vi "Calibration.vi"() -> ()   [LabVIEW 2013]
uses:
  lib/Calibration/Actuator Controls.ctl
  lib/Apps/On Off Button.ctl
  lib/Calibration/Calibration Readings.ctl
  lib/Calibration/CalibrationRampState.ctl
  lib/Calibration/SquareWaveRampState.ctl
  lib/Data Access Objects/Autobalance/Autobalance Control Parameters.ctl
  lib/Calibration/Cal Autobalance State.ctl
  lib/Apps/Yes No Button.ctl
  lib/Autobalance/Autobalance Stage.ctl
  lib/Calibration/Cal Autobalance Loop States.ctl
  lib/Autobalance/Autobalance State.ctl
  Test Utilities/DAQ Read Actions.ctl
  lib/Autobalance/Autobalance Status Data.ctl
  lib/Autobalance/Autobalance Data Point.ctl
  lib/Data Access Objects/Metadata/LBCB Number.ctl
  <vilib>/DAQmx/write.llb/DAQmx Write (Analog 1D DBL NChan 1Samp).vi
  <vilib>/DAQmx/miscellaneous.llb/DAQmx Fill In Error Info.vi
panel:
  out "Cal Sensor":dbl[](array[numeric])
  out "Cal Sensor GUI":dbl[](array[numeric]) caption="Cal Sensor"
  out "Servo Error Reading GUI":dbl[](array[numeric])=[-0.045613668785055836, 0.05618794485593462, -0.029714015687887337, -2.1182198949074764, 0.2302475954600103, 0.1361257374672665] caption="Servo Error \nReading"
  out "Load Cell \nReading  GUI":dbl[](array[numeric])=[0.004815892305044922, 0.021102771948247747, 0.11524760557242354, -0.004639114097545322, -0.030749291237820664, 0.2506269888196334] caption="Load Cell \nReading"
  out "LVDT Reading  GUI":dbl[](array[numeric])=[-0.007330159215639922, -0.035690290111210145, 0.0164473634355215, 0.754492764389709, -0.07873676501809232, -0.046523640832661604] caption="LVDT Reading"
  in  "Control Type":enum32{"Set", "Ramp", "Square", "Autobalance"}(tab)=enum."Autobalance"
  in  "Set Control":cluster{"Set":bool, "Actuator Controls":T1} {"Actuator Controls"."Actuator Z2" min=-10.0 max=10.0 step=0.1 scale=-10.0..10.0; "Actuator Controls"."Actuator Z3" min=-10.0 max=10.0 step=0.1 scale=-10.0..10.0; "Actuator Controls"."Actuator X2" min=-10.0 max=10.0 step=0.1 scale=-10.0..10.0; "Actuator Controls"."Actuator Y1" min=-10.0 max=10.0 step=0.1 scale=-10.0..10.0; "Actuator Controls"."Actuator Z1" min=-10.0 max=10.0 step=0.1 scale=-10.0..10.0; "Actuator Controls"."Actuator X1" min=-10.0 max=10.0 step=0.1 scale=-10.0..10.0}
  in  "Ramp Control":T2={"Ramp Time\n(millseconds)"=30.0, "No. of Steps"=100, "Ramp"=FALSE, "Actuator Controls"={"Actuator X1"=0.0, "Actuator X2"=0.0, "Actuator Y1"=0.0, "Actuator Z1"=0.0, "Actuator Z2"=0.0, "Actuator Z3"=0.0}} {"Actuator Controls"."Actuator Z2" min=-10.0 max=10.0 step=0.1 scale=-10.0..10.0; "Actuator Controls"."Actuator Z3" min=-10.0 max=10.0 step=0.1 scale=-10.0..10.0; "Actuator Controls"."Actuator X2" min=-10.0 max=10.0 step=0.1 scale=-10.0..10.0; "Actuator Controls"."Actuator Y1" min=-10.0 max=10.0 step=0.1 scale=-10.0..10.0; "Actuator Controls"."Actuator Z1" min=-10.0 max=10.0 step=0.1 scale=-10.0..10.0; "Actuator Controls"."Actuator X1" min=-10.0 max=10.0 step=0.1 scale=-10.0..10.0}
  in  "Ramp State":T3
  out "Number of Samples":i32=1031
  out "High Square":dbl=0.0003013857302646694
  out "Low Square":dbl=0.0003106730021702475
  in  "Square State":T4
  in  "Square Control":T5={"Hold Time\n(milliseconds)"=12000, "No. of\n Iterations"=20, "Run"=FALSE, "Actuator Controls"={"Actuator X1"=0.0, "Actuator X2"=0.0, "Actuator Y1"=0.0, "Actuator Z1"=0.2, "Actuator Z2"=0.0, "Actuator Z3"=0.0}} {"Actuator Controls"."Actuator Z2" min=-10.0 max=10.0 step=0.1 scale=-10.0..10.0; "Actuator Controls"."Actuator Z3" min=-10.0 max=10.0 step=0.1 scale=-10.0..10.0; "Actuator Controls"."Actuator X2" min=-10.0 max=10.0 step=0.1 scale=-10.0..10.0; "Actuator Controls"."Actuator Y1" min=-10.0 max=10.0 step=0.1 scale=-10.0..10.0; "Actuator Controls"."Actuator Z1" min=-10.0 max=10.0 step=0.1 scale=-10.0..10.0; "Actuator Controls"."Actuator X1" min=-10.0 max=10.0 step=0.1 scale=-10.0..10.0}
  in  "course":u32=2500
  in  "fine":i32=100
  out "Square Index":i32=3
  in  "Autobalance":bool
  in  "Error Tolerance":dbl=0.005
  out "Cal Autobalance State":T6
  in  "Autobalance \nControl Parameters":T9={"Number of Samples"=30, "Delay After Cmd"=50, "Maximum Command"=8.5, "1/4 Linear Range"=0.2}
  out "Autobalance Loop State":T10 caption="State"
  out "Autobalance State Out":T11
  in  "Zoom Type":T12(ring)=enum."Lower Edge"
  in  "Restore":bool
  in  "Zoom In":bool
  in  "Readings":T13
  in  "Actuator":i32(listbox)=3
  out "Readings":T14(graph)={"Average[0]"=-0.007330159215639922, "Average[1]"=-0.035690290111210145, "Average[2]"=0.0164473634355215, "Average[3]"=0.754492764389709, "Average[4]"=-0.07873676501809232, "Average[5]"=-0.046523640832661604, "Average[6]"=0.0, "Average[7]"=0.0, "Average[8]"=0.0}
  in  "Logging":T15
  out "Command \nVoltage":dbl[](array[numeric])
  in  "Log File Path":path=path "C:/Documents and Settings/mbletzin/Desktop/CalVolts.txt"
  out "Control Voltage":dbl[](array[numeric])
  in  "rate":dbl=100.0
  in  "samples per \nchannel":i32=30 caption="samples per channel"
  out "Servo Error Reading":dbl[](array[numeric])=[-0.045067125531769704, 0.05668122915132235, -0.02948210200083762, -2.1175081409061565, 0.230346235434936, 0.13661629420139546]
  in  "Command Voltage Task":refnum<k21>="Command Voltage"
  in  "Readings Task":refnum<k21>="All Readings"
  out "Read error out":errorcluster
  out "Write error out":errorcluster
  in  "Read error in (no error)":errorcluster
  out "Load Cell \nReading":dbl[](array[numeric])=[0.004986511517158722, 0.021102771948253347, 0.11523427762419364, -0.004596456436788376, -0.03101586222110612, 0.24965138792681876]
  out "LVDT Reading":dbl[](array[numeric])=[-0.007431458122470593, -0.03581289816268755, 0.016426039174719534, 0.7542049018799244, -0.07857947210067343, -0.04675023078564846]
  in  "Quit":bool
  # "LBCB CALIBRATION PROGRAM"
  # "Sample Window Size"
  # "msec"
  # "deleted\nsamples"
  # "Is Balanced"
  # "State"
  # "(Volts)"
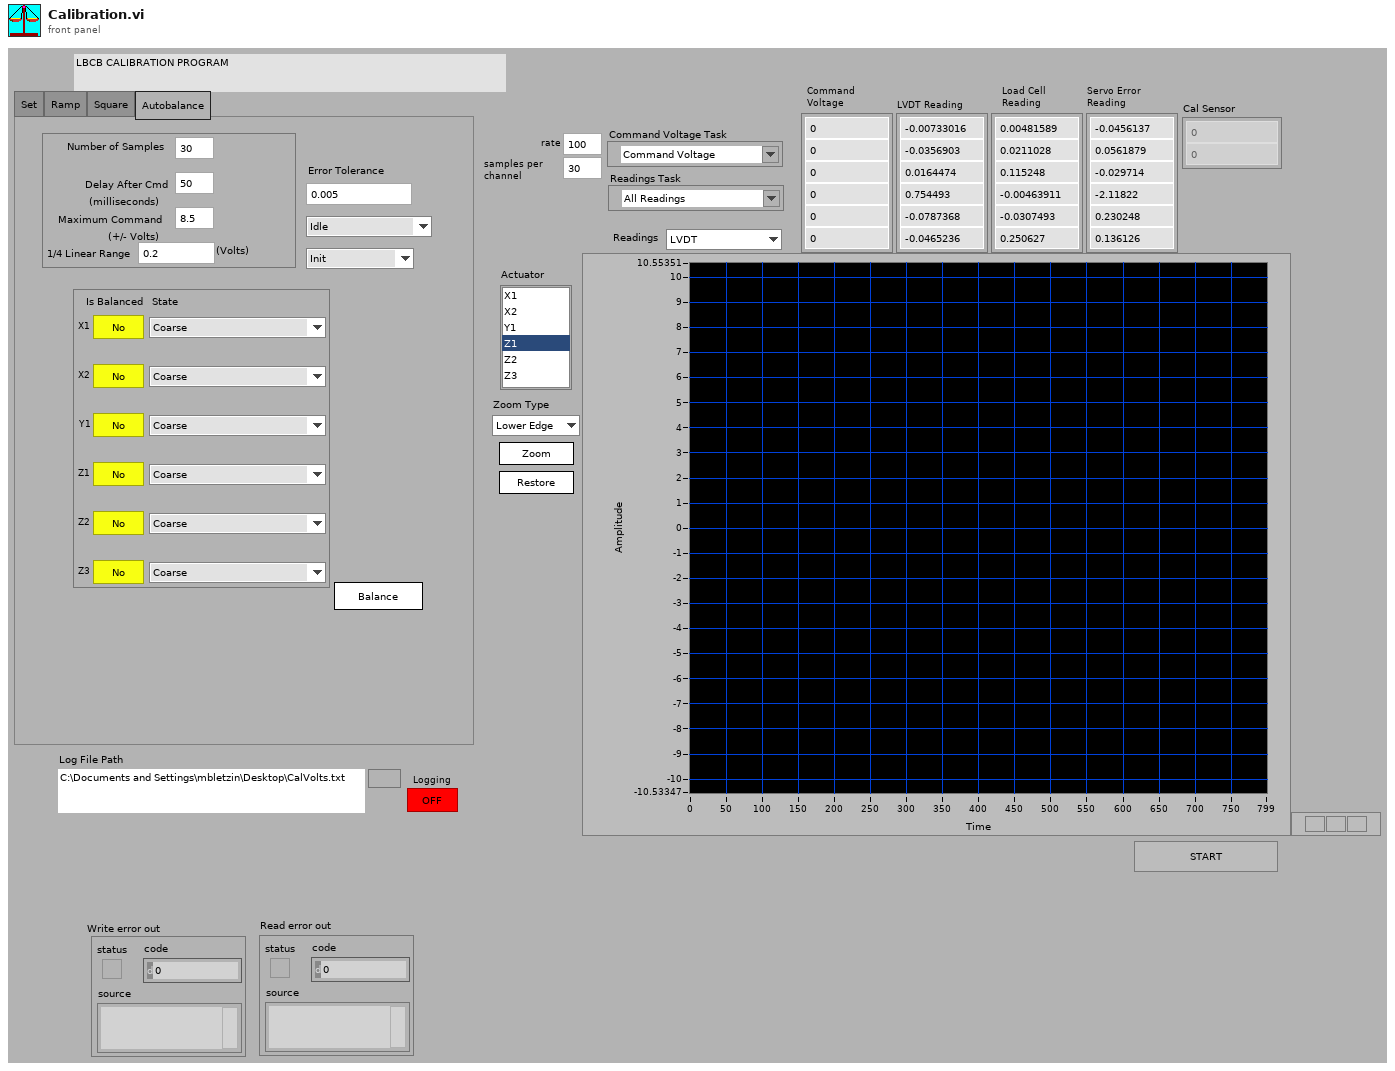
[diagram p1: front panel]
types:
  T1 = typedef "Actuator Controls.ctl" = cluster{"Actuator X1":dbl, "Actuator X2":dbl, "Actuator Y1":dbl, "Actuator Z1":dbl, "Actuator Z2":dbl, "Actuator Z3":dbl}
  T2 = cluster{"Ramp Time\n(millseconds)":dbl, "No. of Steps":i32, "Ramp":bool, "Actuator Controls":T1}
  T3 = typedef "CalibrationRampState.ctl" = enum16{"Idle", "Start Ramp", "Ramping", "Stopping"}
  T4 = typedef "SquareWaveRampState.ctl" = enum16{"Idle", "Start Wave", "High", "Low", "Stop"}
  T5 = cluster{"Hold Time\n(milliseconds)":i32, "No. of\n Iterations":i32, "Run":bool, "Actuator Controls":T1}
  T6 = typedef "Cal Autobalance State.ctl" = cluster{"X1 IsBalanced":T7, "X1 State":T8, "X2 IsBalanced":T7, "X2 State":T8, "Y1 IsBalanced":T7, "Y1 State":T8, "Z1 IsBalanced":T7, "Z1 State":T8, "Z2 IsBalanced":T7, "Z2 State":T8, "Z3 IsBalanced":T7, "Z3 State":T8}
  T7 = typedef "Yes No Button.ctl" = bool
  T8 = typedef "Autobalance Stage.ctl" = enum16{"Coarse", "Fine", "Backing Up", "Done"}
  T9 = typedef "Autobalance Control Parameters.ctl" = cluster{"Number of Samples":i32, "Delay After Cmd":i32, "Maximum Command":dbl, "1/4 Linear Range":dbl}
  T10 = typedef "Cal Autobalance Loop States.ctl" = enum16{"Idle", "Start Balancing", "Balancing", "Stop"}
  T11 = typedef "Autobalance State.ctl" = enum16{"Init", "Send High ", "Wait High", "Read High Start", "Read High", "Send Low", "Wait Low", "Read Low Start", "Read Low", "Publish", "Calculate", "Done"}
  T12 = enum16{"Full", "Upper Half", "Upper Edge", "Lower Half", "Lower Edge"}
  T13 = typedef "Calibration Readings.ctl" = enum16{"LVDT", "Load Cell", "Servo Errors"}
  T14 = cluster{"Average[0]":dbl, "Average[1]":dbl, "Average[2]":dbl, "Average[3]":dbl, "Average[4]":dbl, "Average[5]":dbl, "Average[6]":dbl, "Average[7]":dbl, "Average[8]":dbl}
  T15 = typedef "On Off Button.ctl" = bool
  T16 = enum8{"Enabled", "Disabled", "Disabled and Grayed Out"}
  T17 = typedef "DAQ Read Actions.ctl" = enum16{"Start", "Read", "Stop"}
  T18 = typedef "Autobalance Status Data.ctl" = cluster{"IsBalanced":T7, "Autobalance Stage":T8, "High":T19, "Low":T19, "Balanced \nCmd":dbl}
  T19 = typedef "Autobalance Data Point.ctl" = cluster{"cCmd":dbl, "cServo":dbl, "pCmd":dbl, "pServo":dbl}
  T20 = typedef "LBCB Number.ctl" = enum16{"LBCB1", "LBCB2"}
  T21 = cluster{"Average[0]":dbl, "Average[1]":dbl, "Average[2]":dbl, "Average[3]":dbl, "Average[4]":dbl, "Average[5]":dbl, "Average[6]":dbl, "Average[7]":dbl, "Average[8]":dbl}[]
  T22 = enum16{"open", "replace", "create", "open or create", "replace or create", "replace or create with confirmation"}
  T23 = cluster{"Servo Error Reading[0]":dbl, "Servo Error Reading[1]":dbl, "Servo Error Reading[2]":dbl, "Servo Error Reading[3]":dbl, "Servo Error Reading[4]":dbl, "Servo Error Reading[5]":dbl, "Servo Error Reading[6]":dbl, "Servo Error Reading[7]":dbl, "Servo Error Reading[8]":dbl}
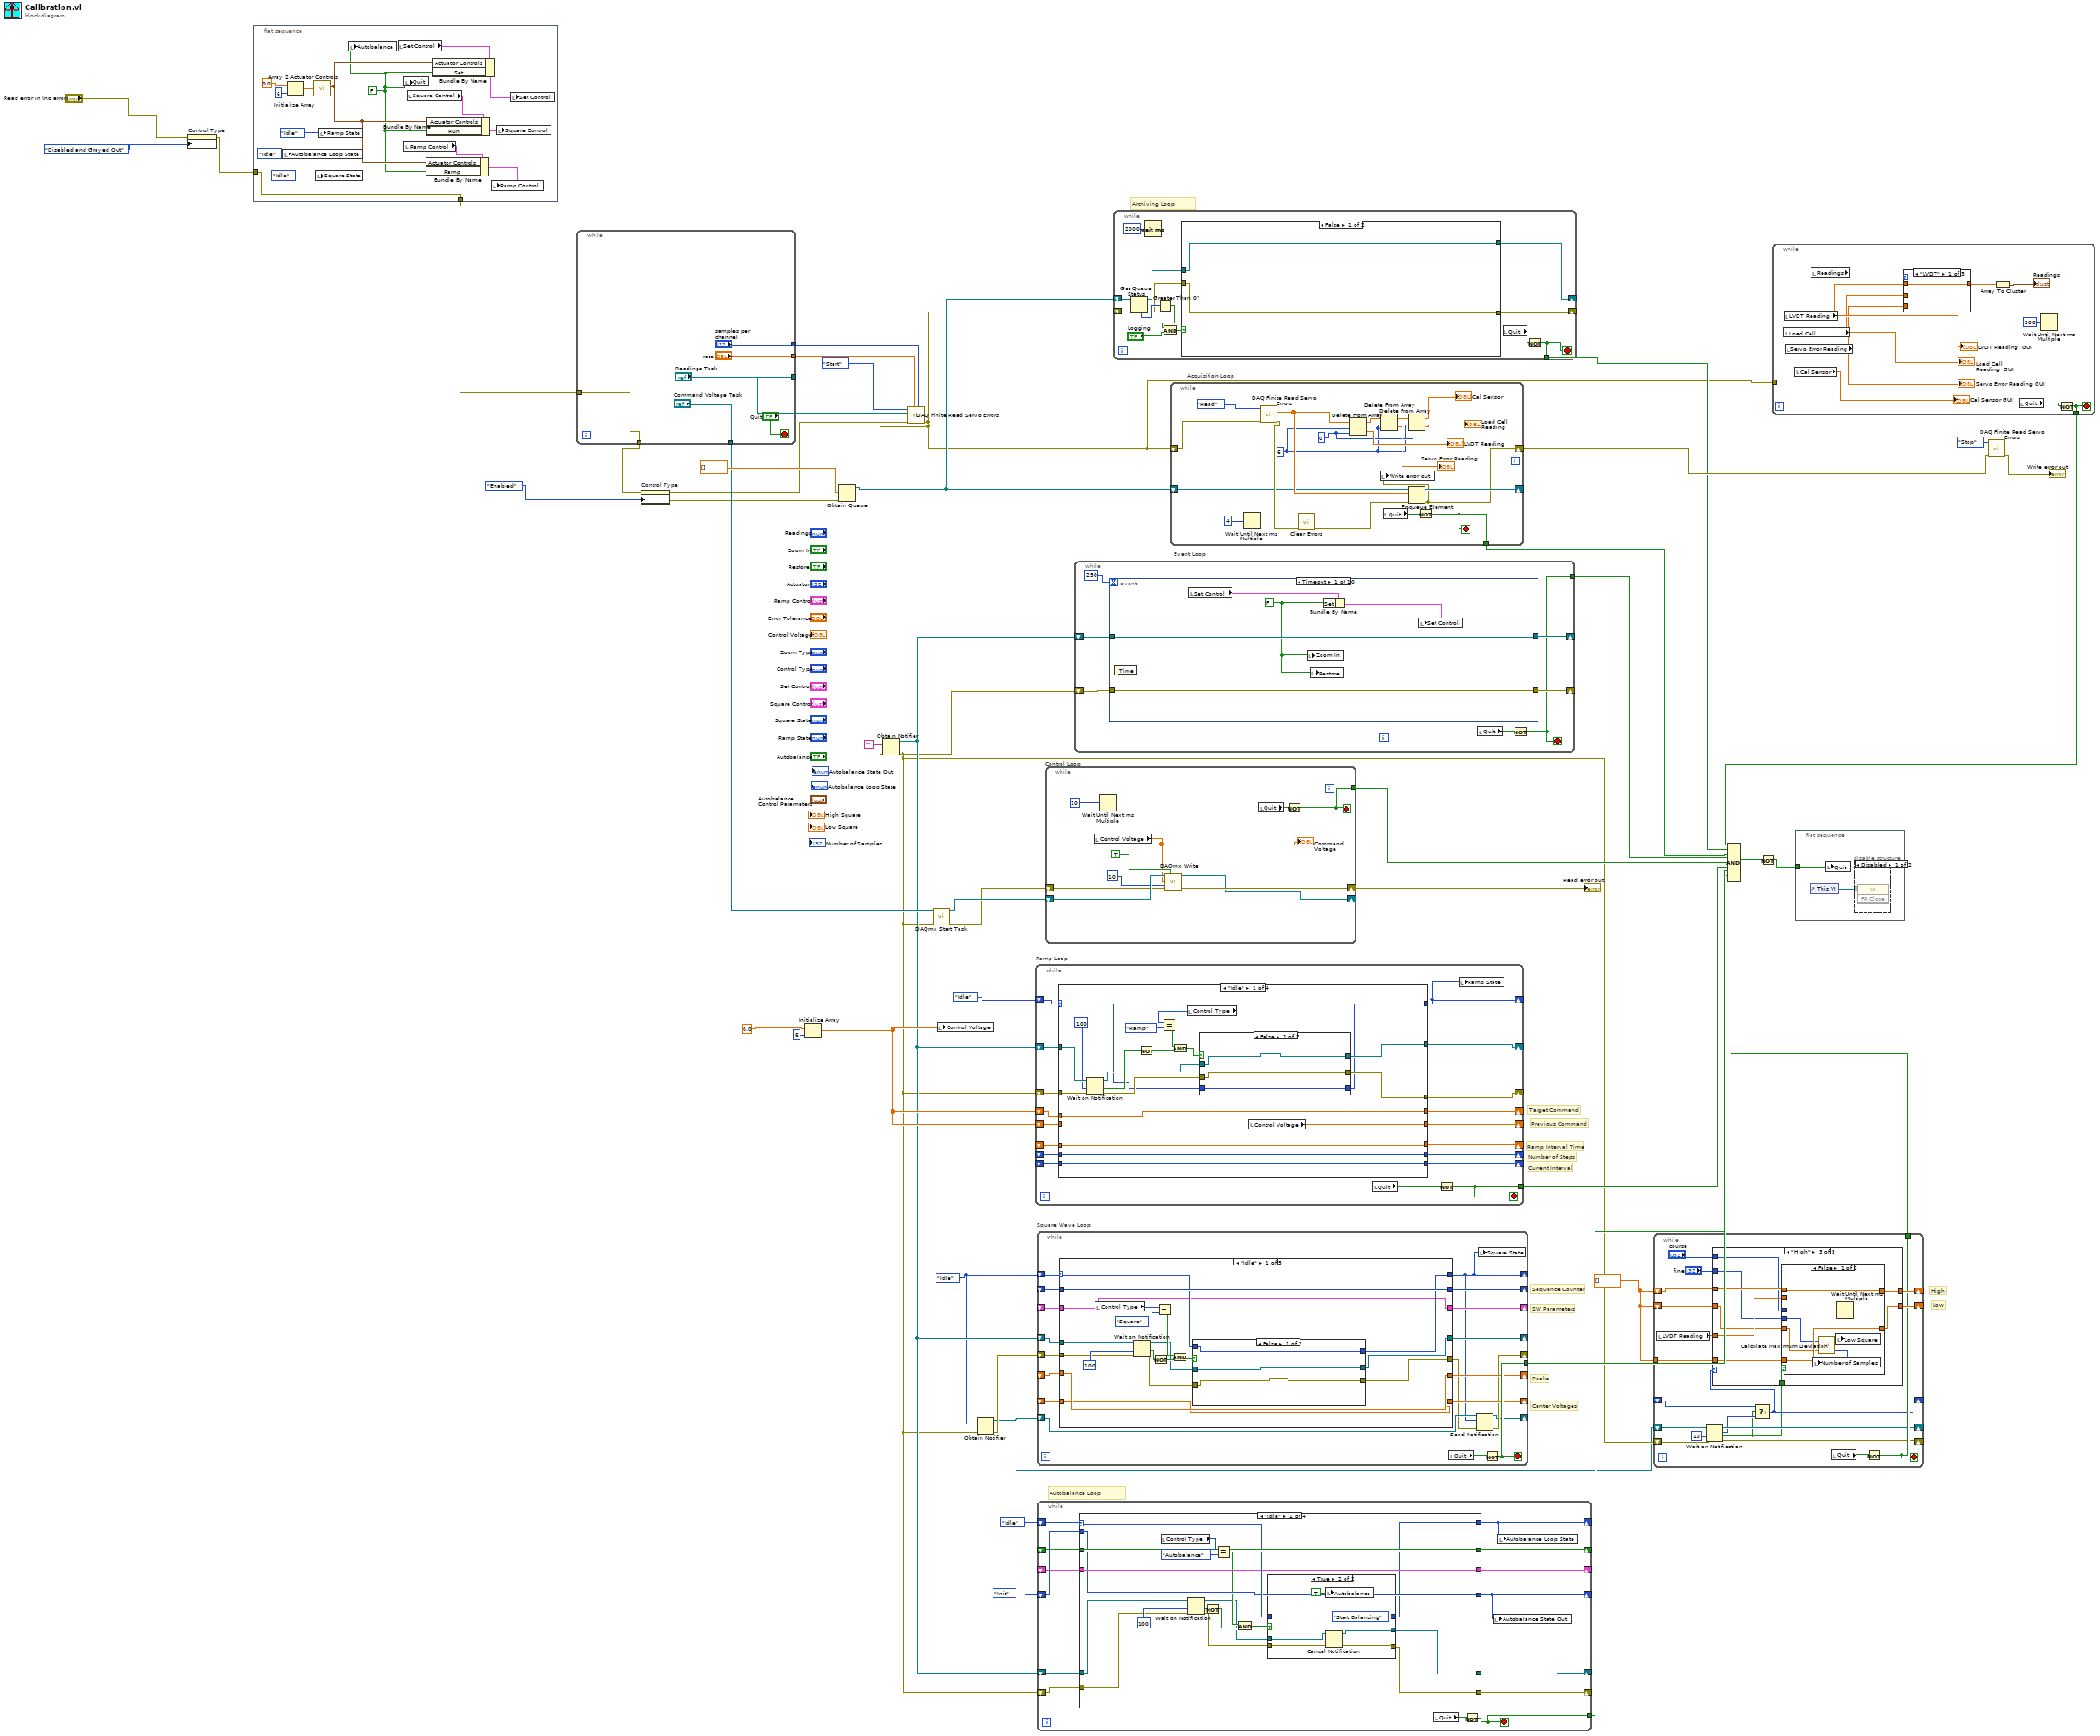
[diagram p0: block diagram]
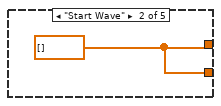
[diagram p5: hidden frame]
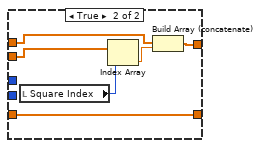
[diagram p6: hidden frame]
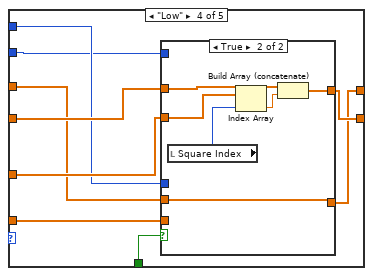
[diagram p7: hidden frame]
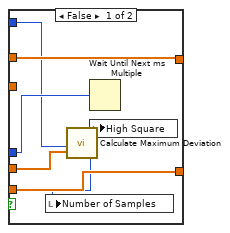
[diagram p8: hidden frame]
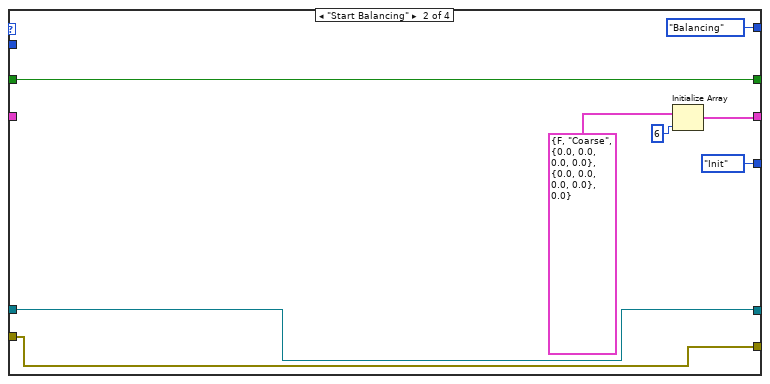
[diagram p11: hidden frame]
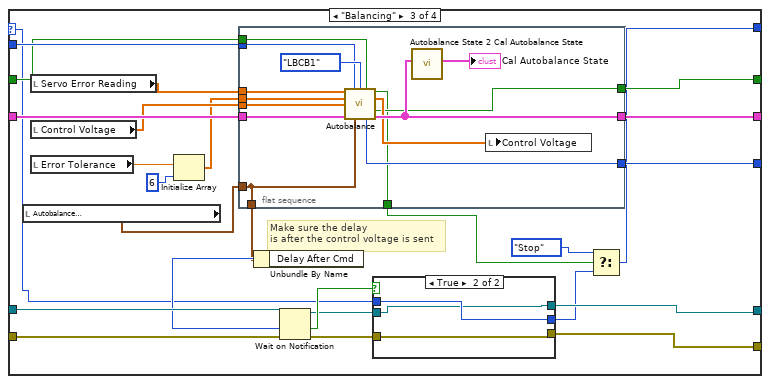
[diagram p12: hidden frame]
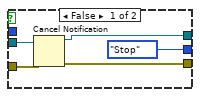
[diagram p13: hidden frame]
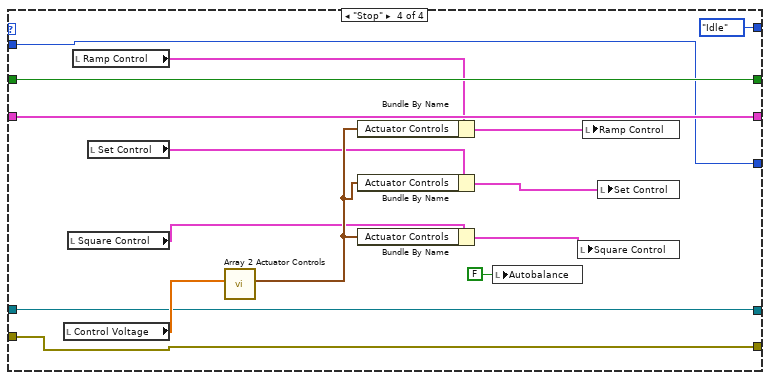
[diagram p14: hidden frame]
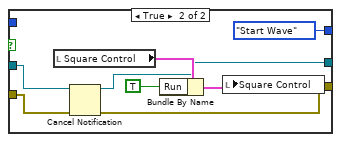
[diagram p15: hidden frame]
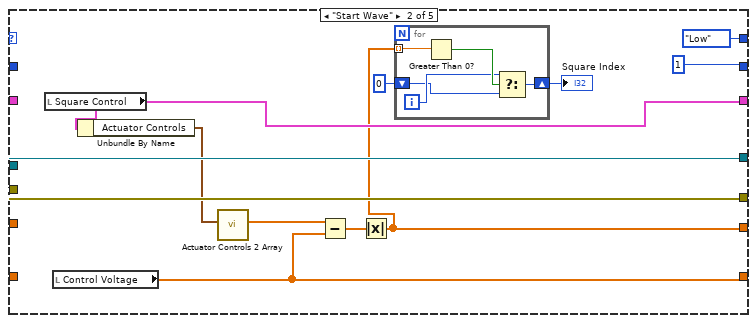
[diagram p16: hidden frame]
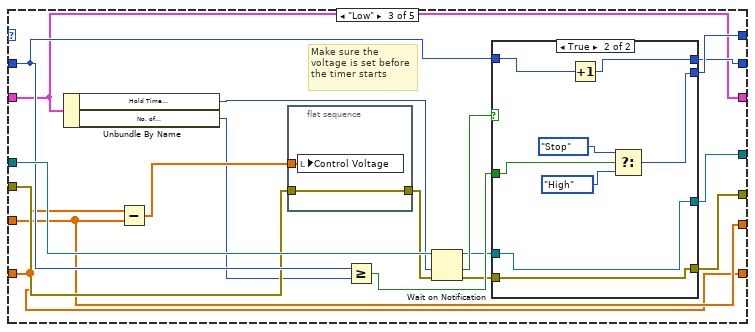
[diagram p17: hidden frame]
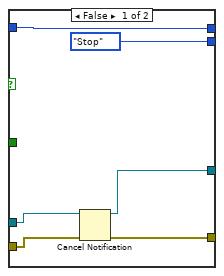
[diagram p18: hidden frame]
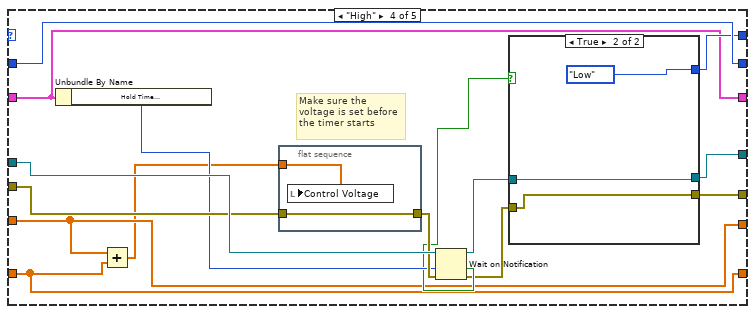
[diagram p19: hidden frame]
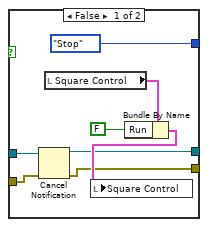
[diagram p20: hidden frame]
diagram:
  w5 = dbl[] []
  w4 = SquareWaveRampState."Idle" ("Square State")
  # "Low"
  # "High"
  # "Autobalance Loop"
  # "Peaks"
  # "Center Voltages"
  # "Archiving Loop"
  # "SW Parameters"
  # "Sequence Counter"
  # "Previous Command"
  # "Target Command"
  # "Ramp Interval Time"
  # "Number of Steps"
  # "Current Interval"
  n1 = property on="Control Type" class="TabCtl (strict)"(error in="Read error in (no error)", "DisabledEnum"=T16."Disabled and Grayed Out" ("Disabled")) -> (error out=w12:errorcluster)  [unwired: 1 in, 1 out]
  n2 = flat-sequence {
    tunnel: w12 -> [w50]
    tunnel: [w50] -> w15
    frame #0 {
      w46 = FALSE
      n3 = local write "Autobalance Loop State"(Cal_Autobalance_Loop_States."Idle" ("Autobalance Loop State")) -> ()
      n4 = Initialize Array(0.0 ("element"), 6 ("dimension size")) -> (w58:dbl[])
      n5 = call "Array 2 Actuator Controls.vi"("Array"=w58) -> ("Actuator Controls"=w51:T1)  [unwired: 10 in]
      n6 = local write "Square State"(SquareWaveRampState."Idle" ("Square State")) -> ()
      n7 = local write "Ramp State"(CalibrationRampState."Idle" ("Ramp State")) -> ()
      n8 = local write "Autobalance"(w46) -> ()
      n9 = local read "Set Control"() -> (w54:cluster{"Set":bool, "Actuator Controls":T1})
      n10 = local write "Quit"(w46) -> ()
      n11 = local read "Ramp Control"() -> (w52:T2)
      n12 = local read "Square Control"() -> (w56:T5)
      n13 = Bundle By Name(cluster=w52, "Actuator Controls"=w51, "Ramp"=w46) -> (w53:T2)
      n14 = Bundle By Name(cluster=w56, "Actuator Controls"=w51, "Run"=w46) -> (w57:T5)
      n15 = Bundle By Name(cluster=w54, "Actuator Controls"=w51, "Set"=w46) -> (w55:cluster{"Set":bool, "Actuator Controls":T1})
      n16 = local write "Ramp Control"(w53) -> ()
      n17 = local write "Square Control"(w57) -> ()
      n18 = local write "Set Control"(w55) -> ()
    }
  }
  n19 = while {
    tunnel: [w61] -> w11
    tunnel: ["samples per \nchannel"] -> w26
    tunnel: ["rate"] -> w25
    tunnel: ["Readings Task"] -> w24
    tunnel: ["Command Voltage Task"] -> w23
    tunnel: w15 -> [w61]
    stop <- "Quit" stop-if-true
  }
  n20 = property on="Control Type" class="TabCtl (strict)"(error in=w11, "DisabledEnum"=T16."Enabled" ("Disabled")) -> (error out=w10:errorcluster)  [unwired: 1 in, 1 out]
  n21 = Initialize Array(0.0 ("element"), 6 ("dimension size")) -> (w22:dbl[])
  n22 = Obtain Queue(element data type=dbl[] [], error in (no error)=w10) -> (queue out=w30:refnum<queue>)  [unwired: 3 in, 2 out]
  n23 = call "DAQ Finite Read Servo Errors.vi"("samples per channel"=w26, "rate"=w25, "error in"=w10, "task/channels in"=w24, "Action"=DAQ_Read_Actions."Start") -> ("error out"=w8:errorcluster)  [unwired: 6 out]
  n24 = Obtain Notifier(notification data type="", error in (no error)=w8) -> (notifier out=w16:refnum<notifier>, error out=w3:errorcluster)  [unwired: 2 in, 1 out]
  n25 = call <vilib>:"DAQmx Start Task.vi"("task/channels in"=w23, "error in"=w3) -> ("task out"=w45:refnum<k21>, "error out"=w20:errorcluster)  [unwired: 12 out]
  n26 = local write "Control Voltage"(w22) -> ()
  n27 = Obtain Notifier(notification data type=w4, error in (no error)=w3) -> (notifier out=w1:refnum<notifier>, error out=w2:errorcluster)  [unwired: 2 in, 1 out]
  n28 = while "Ramp Loop" {
    shift-right: [w67] -> _
    shift-left: CalibrationRampState."Idle" ("Ramp State") -> [w84]
    shift-right: [w81] -> _
    shift-left: w16 -> [w83]
    shift-right: [w80] -> _
    shift-left: w3 -> [w82]
    shift-right: [w79] -> _
    shift-left: _ -> [w71]
    shift-right: [w77] -> _
    shift-left: _ -> [w72]
    shift-right: [w78] -> _
    shift-left: _ -> [w73]
    shift-right: [w76] -> _
    shift-left: w22 -> [w74]
    shift-right: [w75] -> _
    shift-left: w22 -> [w70]
    tunnel: [w68] -> w32
    stop <- w68 stop-if-true
    n29 = case shown="\"Idle\"" w84 {
      selector: w84 -> [w85 _ w139 _]
      tunnel: w83 -> [w104 w125 w138 w173]
      tunnel: w82 -> [w103 w126 w134 w168]
      tunnel: [w87 w125 w132 w173] -> w81
      tunnel: [w88 w126 w128 w168] -> w80
      tunnel: [w86 CalibrationRampState."Ramping" ("f") w129 CalibrationRampState."Idle" ("f")] -> w67
      tunnel: [w99 w122 w147 w171] -> w79
      tunnel: [w97 0 w146 w169] -> w78
      tunnel: [w98 w120 w140 w170] -> w77
      tunnel: [w101 w119 w136 w174] -> w76
      tunnel: [w100 w116 w137 w175] -> w75
      tunnel: w74 -> [_ w119 w136 _]
      tunnel: w73 -> [w97 _ w141 w169]
      tunnel: w72 -> [w98 _ w140 w170]
      tunnel: w71 -> [w99 _ w147 w171]
      tunnel: w70 -> [w100 _ w137 w175]
      frame "Idle" {
        n30 = Wait on Notification(notifier=w104, timeout in ms (-1)=100, error in (no error)=w103) -> (notifier out=w90:refnum<notifier>, timed out?=w96:bool, error out=w89:errorcluster)  [unwired: 1 in, 1 out]
        n31 = Not(x=w96) -> (.not. x?=w91:bool)
        n32 = local read "Control Type"() -> (w95:enum32{"Set", "Ramp", "Square", "Autobalance"})
        n33 = Equal?(x=w95, y=enum32{"Set", "Ramp", "Square", "Autobalance"}."Ramp") -> (x = y?=w93:bool)
        n34 = And(x=w93, y=w91) -> (x .and. y?=w94:bool)
        n35 = case shown="False" w94 {
          tunnel: w90 -> [w107 w112]
          tunnel: w89 -> [w106 w111]
          tunnel: [w106 w109] -> w88
          tunnel: [w107 w110] -> w87
          tunnel: [w105 CalibrationRampState."Start Ramp" ("f")] -> w86
          tunnel: w85 -> [w105 _]
          frame False {
          }
          frame True {
            n36 = local read "Ramp Control"() -> (w115:T2)
            n37 = Bundle By Name(cluster=w115, "Ramp"=TRUE) -> (w114:T2)
            n38 = local write "Ramp Control"(w114) -> ()
            n39 = Cancel Notification(0:w112, 3:w111) -> (8:w110:refnum<notifier>, 11:w109:errorcluster)  [unwired: 1 out]
          }
        }
        n40 = local read "Control Voltage"() -> (w101:dbl[])
      }
      frame "Start Ramp" {
        n41 = local read "Ramp Control"() -> (w118:T2)
        n42 = Unbundle By Name(w118) -> ("Ramp Time\n(millseconds)"=w123:dbl, "No. of Steps"=w120:i32, "Actuator Controls"=w117:T1)
        n43 = call "Actuator Controls 2 Array.vi"("Actuator Controls"=w117) -> ("Array"=w116:dbl[])  [unwired: 10 in]
        n44 = Divide(x=w123, y=w120) -> (x/y=w122:dbl)
      }
      frame "Ramping" {
        n45 = Increment(x=w141) -> (x+1=w146:i32)
        n46 = Subtract(x=w137, y=w136) -> (x-y=w145:dbl[])
        n47 = Less?(x=w140, y=w141) -> (x < y?=w142:bool)
        n48 = Divide(x=w146, y=w140) -> (x/y=w144:dbl)
        n49 = case shown="True" w142 {
          tunnel: w145 -> [w162 _]
          tunnel: w144 -> [w161 _]
          tunnel: [w158 w163] -> w143
          tunnel: w139 -> [w159 _]
          tunnel: [w159 CalibrationRampState."Stopping" ("Ramp State")] -> w127
          tunnel: w137 -> [_ w163]
          tunnel: w136 -> [w157 _]
          frame False {
            n50 = Multiply(x=w162, y=w161) -> (x*y=w160:dbl[])
            n51 = Add(x=w160, y=w157) -> (x+y=w158:dbl[])
          }
          frame True {
          }
        }
        n52 = Multiply(x=w147, y=1000.0) -> (x*y=w135:dbl)
        n53 = local write "Control Voltage"(w143) -> ()
        n54 = Wait on Notification(notifier=w138, timeout in ms (-1)=w135, error in (no error)=w134) -> (notifier out=w133:refnum<notifier>, timed out?=w130:bool, error out=w131:errorcluster)  [unwired: 1 in, 1 out]
        n55 = case shown="True" w130 {
          tunnel: w133 -> [w153 w156]
          tunnel: [w152 w156] -> w132
          tunnel: w131 -> [w150 w154]
          tunnel: [CalibrationRampState."Stopping" ("f") w155] -> w129
          tunnel: [w149 w154] -> w128
          tunnel: w127 -> [_ w155]
          frame False {
            n56 = Cancel Notification(0:w153, 3:w150) -> (8:w152:refnum<notifier>, 11:w149:errorcluster)  [unwired: 1 out]
          }
          frame True {
          }
        }
      }
      frame "Stopping" {
        n57 = local read "Set Control"() -> (w182:cluster{"Set":bool, "Actuator Controls":T1})
        n58 = local read "Ramp Control"() -> (w181:T2)
        n59 = local read "Square Control"() -> (w180:T5)
        n60 = local read "Control Voltage"() -> (w174:dbl[])
        n61 = local read "Ramp Control"() -> (w167:T2)
        n62 = call "Array 2 Actuator Controls.vi"("Array"=w174) -> ("Actuator Controls"=w179:T1)  [unwired: 10 in]
        n63 = Bundle By Name(cluster=w182, "Actuator Controls"=w179) -> (w178:cluster{"Set":bool, "Actuator Controls":T1})
        n64 = Bundle By Name(cluster=w181, "Actuator Controls"=w179) -> (w177:T2)
        n65 = Bundle By Name(cluster=w180, "Actuator Controls"=w179) -> (w176:T5)
        n66 = Bundle By Name(cluster=w167, "Ramp"=FALSE) -> (w166:T2)
        n67 = local write "Square Control"(w176) -> ()
        n68 = local write "Ramp Control"(w177) -> ()
        n69 = local write "Set Control"(w178) -> ()
        n70 = local write "Ramp Control"(w166) -> ()
      }
    }
    n71 = local read "Quit"() -> (w69:bool)
    n72 = Not(x=w69) -> (.not. x?=w68:bool)
    n73 = local write "Ramp State"(w67) -> ()
  }
  n74 = while "Square Wave Loop" {
    tunnel: [w199] -> w21
    shift-right: [w184] -> _
    shift-left: w2 -> [w198]
    shift-right: [w196] -> _
    shift-left: w16 -> [w197]
    shift-right: [w186] -> _
    shift-left: w4 -> [w201]
    shift-right: [w195] -> _
    shift-left: _ -> [w194]
    shift-right: [w193] -> _
    shift-left: _ -> [w191]
    shift-right: [w192] -> _
    shift-left: _ -> [w190]
    shift-right: [w189] -> _
    shift-left: _ -> [w188]
    shift-right: [w183] -> _
    shift-left: w1 -> [w187]
    stop <- w199 stop-if-true
    n75 = case shown="\"Idle\"" w201 {
      selector: w201 -> [w216 _ _ _ _]
      tunnel: w198 -> [w219 w243 w260 w296 w316]
      tunnel: [w202 w243 w249 w283 w316] -> w185
      tunnel: w197 -> [w218 w242 w263 w297 w317]
      tunnel: [w203 w242 w250 w284 w317] -> w196
      tunnel: [w215 SquareWaveRampState."Low" ("Square State") w266 w291 SquareWaveRampState."Idle" ("t")] -> w186
      tunnel: [w217 1 w264 w293 w319] -> w195
      tunnel: w194 -> [w217 _ w262 w293 w319]
      tunnel: [w213 w237 w253 w290 w314] -> w193
      tunnel: [w214 w234 w254 w289 w315] -> w192
      tunnel: w191 -> [w213 _ w253 w290 w314]
      tunnel: w190 -> [w214 _ w254 w289 w315]
      tunnel: [w212 w235 w255 w287 w318] -> w189
      tunnel: w188 -> [w212 _ w255 w287 w325]
      frame "Idle" {
        n76 = local read "Control Type"() -> (w207:enum32{"Set", "Ramp", "Square", "Autobalance"})
        n77 = Wait on Notification(notifier=w218, timeout in ms (-1)=100, error in (no error)=w219) -> (notifier out=w205:refnum<notifier>, timed out?=w210:bool, error out=w204:errorcluster)  [unwired: 1 in, 1 out]
        n78 = Not(x=w210) -> (.not. x?=w206:bool)
        n79 = Equal?(x=w207, y=enum32{"Set", "Ramp", "Square", "Autobalance"}."Square") -> (x = y?=w211:bool)
        n80 = And(x=w211, y=w206) -> (x .and. y?=w209:bool)
        n81 = case shown="False" w209 {
          tunnel: w216 -> [w223 _]
          tunnel: [w223 SquareWaveRampState."Start Wave" ("Square State")] -> w215
          tunnel: w205 -> [w222 w227]
          tunnel: w204 -> [w221 w226]
          tunnel: [w222 w225] -> w203
          tunnel: [w221 w224] -> w202
          frame False {
          }
          frame True {
            n82 = local read "Square Control"() -> (w231:T5)
            n83 = Cancel Notification(0:w227, 3:w226) -> (8:w225:refnum<notifier>, 11:w224:errorcluster)  [unwired: 1 out]
            n84 = Bundle By Name(cluster=w231, "Run"=TRUE) -> (w230:T5)
            n85 = local write "Square Control"(w230) -> ()
          }
        }
      }
      frame "Start Wave" {
        n86 = local read "Square Control"() -> (w235:T5)
        n87 = local read "Control Voltage"() -> (w237:dbl[])
        n88 = Unbundle By Name(w235) -> ("Actuator Controls"=w239:T1)
        n89 = call "Actuator Controls 2 Array.vi"("Actuator Controls"=w239) -> ("Array"=w238:dbl[])  [unwired: 10 in]
        n90 = Subtract(x=w238, y=w237) -> (x-y=w236:dbl[])
        n91 = Absolute Value(x=w236) -> (abs(x)=w234:dbl[])
        n92 = for {
          tunnel: w234 -> [w248] mode=indexing
          shift-right: [w247] -> w232
          shift-left: 0 -> [w244]
          i -> [w245]
          n93 = Greater Than 0?(x=w248) -> (x > 0?=w246:bool)
          n94 = Select(t=w245, s=w246, f=w244) -> (s? t:f=w247:i32)
        }
        "Square Index" <- w232
      }
      frame "Low" {
        # "Make sure the \nvoltage is set before\nthe timer starts"
        n95 = Unbundle By Name(w255) -> ("Hold Time\n(milliseconds)"=w256:i32, "No. of\n Iterations"=w257:i32)
        n96 = Subtract(x=w253, y=w254) -> (x-y=w258:dbl[])
        n97 = flat-sequence {
          tunnel: w260 -> [w268]
          tunnel: [w268] -> w259
          tunnel: w258 -> [w267]
          frame #0 {
            n98 = local write "Control Voltage"(w267) -> ()
          }
        }
        n99 = Greater Or Equal?(x=w262, y=w257) -> (x >= y?=w265:bool)
        n100 = Wait on Notification(notifier=w263, timeout in ms (-1)=w256, error in (no error)=w259) -> (notifier out=w252:refnum<notifier>, timed out?=w261:bool, error out=w251:errorcluster)  [unwired: 1 in, 1 out]
        n101 = case shown="True" w261 {
          tunnel: [SquareWaveRampState."Stop" ("t") w275] -> w266
          tunnel: w265 -> [_ w276]
          tunnel: w262 -> [w274 w282]
          tunnel: [w274 w281] -> w264
          tunnel: w252 -> [w272 w280]
          tunnel: w251 -> [w271 w279]
          tunnel: [w270 w280] -> w250
          tunnel: [w269 w279] -> w249
          frame False {
            n102 = Cancel Notification(0:w272, 3:w271) -> (8:w270:refnum<notifier>, 11:w269:errorcluster)  [unwired: 1 out]
          }
          frame True {
            n103 = Increment(x=w282) -> (x+1=w281:i32)
            n104 = Select(t=SquareWaveRampState."Stop", s=w276, f=SquareWaveRampState."High" ("t")) -> (s? t:f=w275:T4)
          }
        }
      }
      frame "High" {
        # "Make sure the \nvoltage is set before\nthe timer starts"
        n105 = Unbundle By Name(w287) -> ("Hold Time\n(milliseconds)"=w294:i32)
        n106 = Add(x=w289, y=w290) -> (x+y=w288:dbl[])
        n107 = flat-sequence {
          tunnel: w296 -> [w310]
          tunnel: [w310] -> w295
          tunnel: w288 -> [w309]
          frame #0 {
            n108 = local write "Control Voltage"(w309) -> ()
          }
        }
        n109 = Wait on Notification(notifier=w297, timeout in ms (-1)=w294, error in (no error)=w295) -> (notifier out=w286:refnum<notifier>, timed out?=w292:bool, error out=w285:errorcluster)  [unwired: 1 in, 1 out]
        n110 = case shown="True" w292 {
          tunnel: [SquareWaveRampState."Stop" ("t") SquareWaveRampState."Low" ("t")] -> w291
          tunnel: w286 -> [w301 w307]
          tunnel: w285 -> [w300 w306]
          tunnel: [w299 w307] -> w284
          tunnel: [w298 w306] -> w283
          frame False {
            n111 = Cancel Notification(0:w301, 3:w300) -> (8:w299:refnum<notifier>, 11:w298:errorcluster)  [unwired: 1 out]
            n112 = local read "Square Control"() -> (w304:T5)
            n113 = Bundle By Name(cluster=w304, "Run"=FALSE) -> (w302:T5)
            n114 = local write "Square Control"(w302) -> ()
          }
          frame True {
          }
        }
      }
      frame "Stop" {
        n115 = local read "Ramp Control"() -> (w324:T2)
        n116 = local read "Set Control"() -> (w322:cluster{"Set":bool, "Actuator Controls":T1})
        n117 = local read "Square Control"() -> (w313:T5)
        n118 = call "Array 2 Actuator Controls.vi"("Array"=w314) -> ("Actuator Controls"=w326:T1)  [unwired: 10 in]
        n119 = Bundle By Name(cluster=w325, "Actuator Controls"=w326) -> (w318:T5)
        n120 = Bundle By Name(cluster=w324, "Actuator Controls"=w326) -> (w323:T2)
        n121 = Bundle By Name(cluster=w322, "Actuator Controls"=w326) -> (w321:cluster{"Set":bool, "Actuator Controls":T1})
        n122 = Bundle By Name(cluster=w313, "Run"=FALSE) -> (w311:T5)
        n123 = local write "Control Voltage"(w314) -> ()
        n124 = local write "Square Control"(w311) -> ()
        n125 = local write "Square Control"(w318) -> ()
        n126 = local write "Ramp Control"(w323) -> ()
        n127 = local write "Set Control"(w321) -> ()
      }
    }
    n128 = local read "Quit"() -> (w200:bool)
    n129 = Send Notification(notification=w186, notifier=w187, error in (no error)=w185) -> (notifier out=w183:refnum<notifier>, error out=w184:errorcluster)
    n130 = local write "Square State"(w186) -> ()
    n131 = Not(x=w200) -> (.not. x?=w199:bool)
  }
  n132 = while {
    shift-right: [w327] -> _
    shift-left: Cal_Autobalance_Loop_States."Idle" ("Square State") -> [w340]
    shift-right: [w338] -> _
    shift-left: _ -> [w339]
    shift-right: [w328] -> _
    shift-left: Autobalance_State."Init" ("Autobalance State Out") -> [w337]
    shift-right: [w336] -> _
    shift-left: _ -> [w335]
    shift-right: [w330] -> _
    shift-left: w3 -> [w332]
    shift-right: [w331] -> _
    shift-left: w16 -> [w333]
    tunnel: [w329] -> w17
    stop <- w329 stop-if-true
    n133 = case shown="\"Idle\"" w340 {
      selector: w340 -> [w352 _ w378 _]
      tunnel: w339 -> [w357 _ w400 w436]
      tunnel: [w357 w373 w399 w436] -> w338
      tunnel: [w351 Autobalance_State."Init" ("Autobalance State Out") w398 w435] -> w328
      tunnel: w337 -> [w351 _ w397 w435]
      tunnel: [w358 w371 w392 w437] -> w336
      tunnel: w335 -> [w358 w371 w391 w437]
      tunnel: [w350 Cal_Autobalance_Loop_States."Balancing" ("Square State") w388 Cal_Autobalance_Loop_States."Idle" ("Square State")] -> w327
      tunnel: w333 -> [w355 w369 w387 w426]
      tunnel: w332 -> [w354 w368 w386 w425]
      tunnel: [w342 w369 w381 w426] -> w331
      tunnel: [w341 w368 w380 w425] -> w330
      frame "Idle" {
        n134 = local read "Control Type"() -> (w346:enum32{"Set", "Ramp", "Square", "Autobalance"})
        n135 = Wait on Notification(notifier=w355, timeout in ms (-1)=100, error in (no error)=w354) -> (notifier out=w344:refnum<notifier>, timed out?=w353:bool, error out=w343:errorcluster)  [unwired: 1 in, 1 out]
        n136 = Not(x=w353) -> (.not. x?=w348:bool)
        n137 = Equal?(x=w346, y=enum32{"Set", "Ramp", "Square", "Autobalance"}."Autobalance") -> (x = y?=w349:bool)
        n138 = And(x=w349, y=w348) -> (x .and. y?=w347:bool)
        n139 = case shown="True" w347 {
          tunnel: w352 -> [w361 _]
          tunnel: [w361 Cal_Autobalance_Loop_States."Start Balancing" ("Square State")] -> w350
          tunnel: w344 -> [w360 w365]
          tunnel: w343 -> [w359 w364]
          tunnel: [w360 w363] -> w342
          tunnel: [w359 w362] -> w341
          frame False {
          }
          frame True {
            n140 = local write "Autobalance"(TRUE ("Autobalance")) -> ()
            n141 = Cancel Notification(0:w365, 3:w364) -> (8:w363:refnum<notifier>, 11:w362:errorcluster)  [unwired: 1 out]
          }
        }
      }
      frame "Start Balancing" {
        n142 = Initialize Array(T18 {"IsBalanced"=FALSE, "Autobalance Stage"=enum."Coarse", "High"={"cCmd"=0.0, "cServo"=0.0, "pCmd"=0.0, "pServo"=0.0}, "Low"={"cCmd"=0.0, "cServo"=0.0, "pCmd"=0.0, "pServo"=0.0}, "Balanced \nCmd"=0.0} ("Autobalance Persistant Values Out"), 6 ("dimension size")) -> (w373:T18[])
      }
      frame "Balancing" {
        # "Make sure the delay\nis after the control voltage is sent"
        n143 = local read "Autobalance \nControl Parameters"() -> (w376:T9)
        n144 = local read "Servo Error Reading"() -> (w401:dbl[])
        n145 = local read "Control Voltage"() -> (w396:dbl[])
        n146 = local read "Error Tolerance"() -> (w395:dbl)
        n147 = Initialize Array(w395, 6 ("dimension size")) -> (w394:dbl[])
        n148 = flat-sequence {
          tunnel: w401 -> [w415]
          tunnel: w400 -> [w414]
          tunnel: [w412] -> w399
          tunnel: [w410] -> w398
          tunnel: w397 -> [w409]
          tunnel: w396 -> [w408]
          tunnel: w394 -> [w407]
          tunnel: [w405] -> w392
          tunnel: w391 -> [w404]
          tunnel: [w403] -> w389
          tunnel: w376 -> [w402]
          tunnel: [w402] -> w377
          frame #0 {
            n149 = call "Autobalance.vi"("Servo Errors"=w415, 1:"Autobalance State In"=w409, "LBCB Number"=LBCB_Number."LBCB1", "InitialPosition? In"=w404, "Error Tolerance"=w407, "Command In"=w408, 11:"Autobalance State In"=w414, "Autobalance \nControl Parameters"=w402) -> ("IsBalanced"=w403:T7, "Command Out"=w406:dbl[], "InitialPosition? Out"=w405:T7, 14:"Autobalance State Out"=w410:T11, 15:"Autobalance State Out"=w412:T18[])  [unwired: 3 in]
            n150 = call "Autobalance State 2 Cal Autobalance State.vi"("Autobalance State In"=w412) -> ("Cal Autobalance State"=→"Cal Autobalance State":T6)  [unwired: 10 in]
            n151 = local write "Control Voltage"(w406) -> ()
          }
        }
        n152 = Unbundle By Name(w377) -> ("Delay After Cmd"=w385:i32)
        n153 = Wait on Notification(notifier=w387, timeout in ms (-1)=w385, error in (no error)=w386) -> (notifier out=w383:refnum<notifier>, timed out?=w384:bool, error out=w382:errorcluster)  [unwired: 1 in, 1 out]
        n154 = case shown="True" w384 {
          tunnel: w383 -> [w420 w422]
          tunnel: w382 -> [w419 w421]
          tunnel: [w418 w422] -> w381
          tunnel: [w417 w421] -> w380
          tunnel: [Cal_Autobalance_Loop_States."Stop" ("Square State") w423] -> w379
          tunnel: w378 -> [_ w423]
          frame False {
            n155 = Cancel Notification(0:w420, 3:w419) -> (8:w418:refnum<notifier>, 11:w417:errorcluster)  [unwired: 1 out]
          }
          frame True {
          }
        }
        n156 = Select(t=Cal_Autobalance_Loop_States."Stop" ("Square State"), s=w389, f=w379) -> (s? t:f=w388:T10)
      }
      frame "Stop" {
        n157 = local read "Control Voltage"() -> (w430:dbl[])
        n158 = local read "Square Control"() -> (w431:T5)
        n159 = local read "Ramp Control"() -> (w433:T2)
        n160 = local read "Set Control"() -> (w432:cluster{"Set":bool, "Actuator Controls":T1})
        n161 = call "Array 2 Actuator Controls.vi"("Array"=w430) -> ("Actuator Controls"=w434:T1)  [unwired: 10 in]
        n162 = Bundle By Name(cluster=w433, "Actuator Controls"=w434) -> (w427:T2)
        n163 = Bundle By Name(cluster=w432, "Actuator Controls"=w434) -> (w428:cluster{"Set":bool, "Actuator Controls":T1})
        n164 = Bundle By Name(cluster=w431, "Actuator Controls"=w434) -> (w429:T5)
        n165 = local write "Autobalance"(FALSE ("Autobalance")) -> ()
        n166 = local write "Square Control"(w429) -> ()
        n167 = local write "Ramp Control"(w427) -> ()
        n168 = local write "Set Control"(w428) -> ()
      }
    }
    n169 = local read "Quit"() -> (w334:bool)
    n170 = Not(x=w334) -> (.not. x?=w329:bool)
    n171 = local write "Autobalance State Out"(w328) -> ()
    n172 = local write "Autobalance Loop State"(w327) -> ()
  }
  n173 = while "Control Loop" {
    shift-right: [w445] -> _
    shift-left: w45 -> [w448]
    shift-right: [w446] -> w44
    shift-left: w20 -> [w447]
    tunnel: [w440] -> w39
    stop <- w440 stop-if-true
    n174 = local read "Control Voltage"() -> (w439:dbl[])
    "Command \nVoltage" <- w439
    n175 = Wait Until Next ms Multiple(millisecond multiple=10) -> ()  [unwired: 1 out]
    n176 = call-poly <vilib>:"DAQmx Write.vi"("task/channels in"=w448, "auto start"=TRUE, "data"=w439, "timeout"=10, "error in"=w447) -> ("task out"=w445:refnum<k21>, "error out"=w446:errorcluster)  [unwired: 9 out]
    n177 = local read "Quit"() -> (w441:bool)
    n178 = Not(x=w441) -> (.not. x?=w440:bool)
  }
  "Read error out" <- w44
  n179 = while "Event Loop" {
    tunnel: [w449] -> w43
    shift-right: [w450] -> _
    shift-left: w3 -> [w452]
    shift-right: [w451] -> _
    shift-left: w16 -> [w453]
    stop <- w449 stop-if-true
    n180 = event shown="[0] Timeout" {
      selector: _ -> [_ _ _ _ _ _ _ _ _ _]
      dyn-events: _ -> [_ _ _ _ _ _ _ _ _ _]
      timeout: 250 -> [_ _ _ _ _ _ _ _ _ _]
      tunnel: w453 -> [w460 w466 w488 w500 w519 w550 w555 w557 w584 w625]
      tunnel: w452 -> [w459 w465 w487 w499 w522 w551 w554 w562 w583 w627]
      tunnel: [w460 w464 w486 w498 w518 w550 w555 w557 w584 w625] -> w451
      tunnel: [w459 w463 w485 w497 w521 w551 w554 w558 w580 w626] -> w450
      event Timeout {
        w458 = FALSE ("Set")
        n181 = event-data() -> ()  [unwired: 2 out]
        n182 = local read "Set Control"() -> (w456:cluster{"Set":bool, "Actuator Controls":T1})
        n183 = local write "Zoom In"(w458) -> ()
        n184 = local write "Restore"(w458) -> ()
        n185 = Bundle By Name(cluster=w456, "Set"=w458) -> (w457:cluster{"Set":bool, "Actuator Controls":T1})
        n186 = local write "Set Control"(w457) -> ()
      }
      event "Ramp Control.Ramp": Mouse Down? {
        n187 = event-data() -> ()  [unwired: 2 out]
        n188 = local read "Ramp State"() -> (w462:T3)
        n189 = case shown="\"Ramping\"" w462 {
          tunnel: w466 -> [w471 w476 w479 w482]
          tunnel: w465 -> [w469 w474 w478 w481]
          tunnel: [w468 w473 w479 w482] -> w464
          tunnel: [w467 w472 w478 w481] -> w463
          tunnel: [_ _ TRUE TRUE] -> w461
          frame "Idle" {
            n190 = Send Notification(notification="Start", notifier=w471, error in (no error)=w469) -> (notifier out=w468:refnum<notifier>, error out=w467:errorcluster)
          }
          frame "Ramping" {
            n191 = Send Notification(notification="Stop", notifier=w476, error in (no error)=w474) -> (notifier out=w473:refnum<notifier>, error out=w472:errorcluster)
          }
          frame "Stopping" {
          }
          frame "Start Ramp" {
          }
        }
        n192 = event-data("Discard?"=w461) -> ()  [unwired: 1 in, 1 out]
      }
      event "Control Type": Mouse Down? {
        n193 = event-data() -> ("Button"=w484:u16)  [unwired: 1 out]
        n194 = flat-sequence {
          tunnel: w488 -> [w494]
          tunnel: w487 -> [w493]
          tunnel: [w492] -> w486
          tunnel: [w491] -> w485
          tunnel: w484 -> [w490]
          tunnel: [w490] -> w483
          frame #0 {
            n195 = Cancel Notification(0:w494, 3:w493) -> (8:w492:refnum<notifier>, 11:w491:errorcluster)  [unwired: 1 out]
          }
        }
        n196 = event-data("Button"=w483, "Discard?"=FALSE) -> ()  [unwired: 1 in, 1 out]
      }
      event "Autobalance": Mouse Down? {
        n197 = event-data() -> ()  [unwired: 2 out]
        n198 = local read "Autobalance Loop State"() -> (w496:T10)
        n199 = case shown="\"Balancing\"" w496 {
          tunnel: w500 -> [w505 w508 w513 w516]
          tunnel: w499 -> [w503 w507 w511 w515]
          tunnel: [w502 w508 w510 w516] -> w498
          tunnel: [w501 w507 w509 w515] -> w497
          tunnel: [_ TRUE _ TRUE] -> w495
          frame "Idle" {
            n200 = Send Notification(notification="Start", notifier=w505, error in (no error)=w503) -> (notifier out=w502:refnum<notifier>, error out=w501:errorcluster)
          }
          frame "Start Balancing" {
          }
          frame "Balancing" {
            n201 = Send Notification(notification="Stop", notifier=w513, error in (no error)=w511) -> (notifier out=w510:refnum<notifier>, error out=w509:errorcluster)
          }
          frame "Stop" {
          }
        }
        n202 = event-data("Discard?"=w495) -> ()  [unwired: 1 in, 1 out]
      }
      event "Square Control.Run": Mouse Down? {
        n203 = event-data() -> ()  [unwired: 2 out]
        n204 = local read "Square State"() -> (w520:T4)
        n205 = case shown="\"Start Wave\"" w520 {
          tunnel: w519 -> [w527 w532 w537 w540 w543]
          tunnel: w522 -> [w525 w530 w535 w539 w542]
          tunnel: [w524 w529 w534 w540 w543] -> w518
          tunnel: [w523 w528 w533 w539 w542] -> w521
          tunnel: [_ _ _ TRUE TRUE] -> w517
          frame "Idle" {
            n206 = Send Notification(notification="Start", notifier=w527, error in (no error)=w525) -> (notifier out=w524:refnum<notifier>, error out=w523:errorcluster)
          }
          frame "Low" {
            n207 = Send Notification(notification="Stop", notifier=w532, error in (no error)=w530) -> (notifier out=w529:refnum<notifier>, error out=w528:errorcluster)
          }
          frame "High" {
            n208 = Send Notification(notification="Stop", notifier=w537, error in (no error)=w535) -> (notifier out=w534:refnum<notifier>, error out=w533:errorcluster)
          }
          frame "Start Wave" {
          }
          frame "Stop" {
          }
        }
        n209 = event-data("Discard?"=w517) -> ()  [unwired: 1 in, 1 out]
      }
      event "Set Control.Set": Mouse Down {
        n210 = event-data() -> ()  [unwired: 2 out]
        n211 = local read "Set Control"() -> (w552:cluster{"Set":bool, "Actuator Controls":T1})
        n212 = Unbundle By Name(w552) -> ("Actuator Controls"=w545:T1)
        n213 = local read "Square Control"() -> (w546:T5)
        n214 = local read "Ramp Control"() -> (w548:T2)
        n215 = Bundle By Name(cluster=w548, "Actuator Controls"=w545) -> (w547:T2)
        n216 = Bundle By Name(cluster=w546, "Actuator Controls"=w545) -> (w544:T5)
        n217 = call "Actuator Controls 2 Array.vi"("Actuator Controls"=w545) -> ("Array"=w549:dbl[])  [unwired: 10 in]
        n218 = local write "Control Voltage"(w549) -> ()
        n219 = local write "Square Control"(w544) -> ()
        n220 = local write "Ramp Control"(w547) -> ()
      }
      event Value Change {
        n221 = event-data() -> ()  [unwired: 2 out]
        n222 = property on="Readings" class="WFChart (strict)"(error in=w554, "History Data"=T21 []) -> ()  [unwired: 1 in, 2 out]
      }
      event "Actuator": Value Change {
        n223 = event-data() -> ("NewVal"=w565:i32, "OldVal"=w564:i32)  [unwired: 1 out]
        n224 = property on="Readings" class="WFChart (strict)"(error in=w562, "Active Plot"=w564) -> (error out=w563:errorcluster)  [unwired: 1 in, 1 out]
        n225 = property on="Readings" class="WFChart (strict)"(error in=w563, "Plot.Line Width"=u8 0) -> (error out=w560:errorcluster)  [unwired: 1 in, 1 out]
        n226 = property on="Readings" class="WFChart (strict)"(error in=w560, "Active Plot"=w565) -> (error out=w559:errorcluster)  [unwired: 1 in, 1 out]
        n227 = property on="Readings" class="WFChart (strict)"(error in=w559, "Plot.Line Width"=u8 3) -> (error out=w558:errorcluster)  [unwired: 1 in, 1 out]
      }
      event "Zoom In": Mouse Down; "Zoom Type": Value Change {
        n228 = event-data() -> ()  [unwired: 2 out]
        n229 = property on="Readings" class="WFChart (strict)"(error in=w583) -> (error out=w582:errorcluster, "History Data"=w572:T21)  [unwired: 1 in, 1 out]
        n230 = local read "Actuator"() -> (w570:i32)
        n231 = for {
          tunnel: [w587] -> w585 mode=indexing
          tunnel: w572 -> [w586] mode=indexing
          n232 = Cluster To Array(cluster=w586) -> (array=w587:dbl[])
        }
        n233 = Index Array(array=w585, index (col)=w570) -> (element=w571:dbl[])  [unwired: 1 in]
        n234 = Array Max & Min(array=w571) -> (max value=w576:dbl, min value=w575:dbl)  [unwired: 2 out]
        n235 = Subtract(x=w576, y=w575) -> (x-y=w569:dbl)
        n236 = local read "Zoom Type"() -> (w579:T12)
        n237 = Multiply(x=w569, y=0.02) -> (x*y=w577:dbl)
        n238 = Absolute Value(x=w577) -> (abs(x)=w568:dbl)
        n239 = case shown="\"Lower Half\"" w579 {
          tunnel: w568 -> [w589 w597 w605 w614 w621]
          tunnel: w576 -> [w592 w598 w606 w610 w623]
          tunnel: w575 -> [w590 w600 w608 w611 w618]
          tunnel: [w591 w596 w604 w615 w622] -> w574
          tunnel: [w588 w599 w607 w616 w624] -> w573
          tunnel: w569 -> [_ w595 w603 w612 w620]
          tunnel: 0.98 ("y") -> [_ _ w601 _ w617]
          tunnel: 0.5 ("y") -> [_ w593 _ w609 _]
          frame "Full" {
            n240 = Add(x=w592, y=w589) -> (x+y=w591:dbl)
            n241 = Subtract(x=w590, y=w589) -> (x-y=w588:dbl)
          }
          frame "Upper Half" {
            n242 = Multiply(x=w595, y=w593) -> (x*y=w594:dbl)
            n243 = Add(x=w598, y=w597) -> (x+y=w596:dbl)
            n244 = Add(x=w594, y=w600) -> (x+y=w599:dbl)
          }
          frame "Upper Edge" {
            n245 = Multiply(x=w603, y=w601) -> (x*y=w602:dbl)
            n246 = Add(x=w606, y=w605) -> (x+y=w604:dbl)
            n247 = Add(x=w602, y=w608) -> (x+y=w607:dbl)
          }
          frame "Lower Half" {
            n248 = Multiply(x=w612, y=w609) -> (x*y=w613:dbl)
            n249 = Subtract(x=w611, y=w614) -> (x-y=w616:dbl)
            n250 = Subtract(x=w610, y=w613) -> (x-y=w615:dbl)
          }
          frame "Lower Edge" {
            n251 = Multiply(x=w620, y=w617) -> (x*y=w619:dbl)
            n252 = Subtract(x=w618, y=w621) -> (x-y=w624:dbl)
            n253 = Subtract(x=w623, y=w619) -> (x-y=w622:dbl)
          }
        }
        n254 = property on="Readings" class="WFChart (strict)"(error in=w582, "YScale.Maximum"=w574) -> (error out=w581:errorcluster)  [unwired: 1 in, 1 out]
        n255 = property on="Readings" class="WFChart (strict)"(error in=w581, "YScale.Minimum"=w573) -> (error out=w580:errorcluster)  [unwired: 1 in, 1 out]
      }
      event "Restore": Mouse Down {
        n256 = event-data() -> ()  [unwired: 3 out]
        n257 = property on="Readings" class="WFChart (strict)"(error in=w627, "YScale.ScaleFit"=u8 1 ("Y Scale.Scale Fit")) -> (error out=w626:errorcluster)  [unwired: 1 in, 1 out]
      }
    }
    n258 = local read "Quit"() -> (w454:bool)
    n259 = Not(x=w454) -> (.not. x?=w449:bool)
  }
  n260 = while {
    shift-right: [w635] -> _
    shift-left: w30 -> [w641]
    shift-right: [w636] -> _
    shift-left: w8 -> [w640]
    tunnel: [w629] -> w29
    stop <- w629 stop-if-true
    n261 = Get Queue Status(queue=w641, error in (no error)=w640) -> (queue out=w638:refnum<queue>, error out=w637:errorcluster, # elements in queue=w639:i32)  [unwired: 1 in, 5 out]
    n262 = Wait (ms)(milliseconds to wait=u32 2000) -> ()  [unwired: 1 out]
    n263 = Greater Than 0?(x=w639) -> (x > 0?=w631:bool)
    n264 = And(x=w631, y="Logging") -> (x .and. y?=w632:T15)
    n265 = case shown="False" w632 {
      tunnel: w638 -> [w643 w651]
      tunnel: w637 -> [w642 w650]
      tunnel: [w642 w649] -> w636
      tunnel: [w643 w647] -> w635
      frame False {
      }
      frame True {
        n266 = Flush Queue(queue=w651, error in (no error)=w650) -> (queue out=w647:refnum<queue>, remaining elements=w648:cluster{dbl[]}[], error out=w646:errorcluster)
        n267 = for {
          tunnel: w648 -> [w666] mode=indexing
          shift-right: [w663] -> w645
          shift-left: "" -> [w662]
          n268 = Unbundle(w666) -> (w665:dbl[])
          n269 = call "Data 2 Record.vi"("Data"=w665) -> ("Records"=w664:string)  [unwired: 10 in]
          n270 = Concatenate Strings(w662, w664) -> (w663:string)
        }
        n271 = Open/Create/Replace File(file path (use dialog)="Log File Path", error in=w646, operation (0:open)=T22."open or create", access (0:read/write)=enum16{"read/write", "read-only", "write-only"}."write-only") -> (refnum out=w657:refnum<file>, error out=w656:errorcluster)  [unwired: 3 out]
        n272 = Set File Position(refnum=w657, from (0:start)=enum16{"start", "end", "current"}."end", error in=w656) -> (refnum out=w654:refnum<file>, error out=w655:errorcluster)  [unwired: 1 out]
        n273 = Write to Text File(file (use dialog)=w654, text=w645, error in=w655) -> (refnum out=w659:refnum<file>, error out=w660:errorcluster)  [unwired: 2 out]
        n274 = Close File(refnum=w659, error in=w660) -> (error out=w649:errorcluster)  [unwired: 1 out]
      }
    }
    n275 = local read "Quit"() -> (w634:bool)
    n276 = Not(x=w634) -> (.not. x?=w629:bool)
  }
  n277 = while "Acquisition Loop" {
    shift-right: [w672] -> w37
    shift-left: w8 -> [w682]
    tunnel: [w673] -> w41
    shift-right: [w676] -> _
    shift-left: w30 -> [w677]
    stop <- w673 stop-if-true
    w669 = 6
    w670 = 0
    n278 = Wait Until Next ms Multiple(millisecond multiple=4) -> ()  [unwired: 1 out]
    n279 = call "DAQ Finite Read Servo Errors.vi"("error in"=w682, "Action"=DAQ_Read_Actions."Read") -> ("error out"=w681:errorcluster, "Average"=w678:dbl[])  [unwired: 3 in, 5 out]
    n280 = call <vilib>:"Clear Errors.vi"("error in (no error)"=w681) -> ("error out"=w679:errorcluster)  [unwired: 6 out]
    n281 = Delete From Array(array=w678, length=w669, index=w670) -> (deleted portion=→"LVDT Reading":dbl[], array with subset deleted=w683:dbl[])
    n282 = Delete From Array(array=w683, length=w669, index=w669) -> (deleted portion=→"Servo Error Reading":dbl[], array with subset deleted=w674:dbl[])
    n283 = local read "Quit"() -> (w684:bool)
    n284 = Delete From Array(array=w674, length=w669, index=w670) -> (deleted portion=→"Load Cell \nReading":dbl[], array with subset deleted=→"Cal Sensor":dbl[])
    n285 = Enqueue Element(queue=w677, element=w678, error in (no error)=w679) -> (queue out=w676:refnum<queue>, error out=w672:errorcluster)  [unwired: 1 in, 1 out]
    n286 = local write "Write error out"(w672) -> ()
    n287 = Not(x=w684) -> (.not. x?=w673:bool)
  }
  n288 = while {
    shift-right: [w702] -> _
    shift-left: w5 -> [w701]
    shift-right: [w700] -> _
    shift-left: w5 -> [w699]
    shift-right: [w689] -> _
    shift-left: _ -> [w688]
    tunnel: [w698] -> w6
    tunnel: w5 -> [w696]
    shift-right: [w694] -> _
    shift-left: w1 -> [w695]
    shift-right: [w692] -> _
    shift-left: w3 -> [w693]
    stop <- w698 stop-if-true
    n289 = local read "LVDT Reading"() -> (w703:dbl[])
    n290 = Wait on Notification(notifier=w695, timeout in ms (-1)=10, error in (no error)=w693) -> (notifier out=w694:refnum<notifier>, notification=w690:T4, timed out?=w687:bool, error out=w692:errorcluster)  [unwired: 1 in]
    n291 = Select(t=w688, s=w687, f=w690) -> (s? t:f=w689:T4)
    n292 = case shown="\"High\"" w689 {
      tunnel: w703 -> [_ _ w716 w738 _]
      tunnel: [w706 w707 w715 w734 w753] -> w702
      tunnel: w701 -> [w706 _ w714 w732 w753]
      tunnel: [w705 w707 w711 w737 w752] -> w700
      tunnel: w699 -> [w705 _ w713 w736 w752]
      tunnel: "course" -> [_ _ w712 w735 _]
      tunnel: w696 -> [_ _ w710 w733 _]
      tunnel: w687 -> [_ _ w709 w731 _]
      tunnel: "fine" -> [_ _ w708 w730 _]
      frame "Idle" {
      }
      frame "Start Wave" {
        w707 = dbl[] []
      }
      frame "High" {
        n293 = case shown="False" w709 {
          tunnel: w716 -> [_ w729]
          tunnel: [w723 w728] -> w715
          tunnel: w714 -> [w723 w727]
          tunnel: w713 -> [w717 w726]
          tunnel: w712 -> [w721 _]
          tunnel: [w720 w726] -> w711
          tunnel: w710 -> [w720 _]
          tunnel: w708 -> [w719 _]
          frame False {
            n294 = call "Calculate Maximum Deviation.vi"("Sample"=w717, "fine"=w719) -> ("number of samples"=w718:i32, "Outliers"=w722:dbl)
            n295 = local write "Number of Samples"(w718) -> ()
            n296 = local write "Low Square"(w722) -> ()
            n297 = Wait Until Next ms Multiple(millisecond multiple=w721) -> ()  [unwired: 1 out]
          }
          frame True {
            n298 = local read "Square Index"() -> (w724:i32)
            n299 = Index Array(array=w729, index=w724) -> (element=w725:dbl)
            n300 = Build Array (concatenate)(w727, w725) -> (w728:dbl[])
          }
        }
      }
      frame "Low" {
        n301 = case shown="True" w731 {
          tunnel: w738 -> [_ w751]
          tunnel: [w745 w750] -> w737
          tunnel: w736 -> [w745 w749]
          tunnel: w732 -> [w739 w748]
          tunnel: w735 -> [w743 _]
          tunnel: [w742 w748] -> w734
          tunnel: w733 -> [w742 _]
          tunnel: w730 -> [w741 _]
          frame False {
            n302 = call "Calculate Maximum Deviation.vi"("Sample"=w739, "fine"=w741) -> ("number of samples"=w740:i32, "Outliers"=w744:dbl)
            n303 = local write "Number of Samples"(w740) -> ()
            n304 = Wait Until Next ms Multiple(millisecond multiple=w743) -> ()  [unwired: 1 out]
            n305 = local write "High Square"(w744) -> ()
          }
          frame True {
            n306 = local read "Square Index"() -> (w746:i32)
            n307 = Index Array(array=w751, index=w746) -> (element=w747:dbl)
            n308 = Build Array (concatenate)(w749, w747) -> (w750:dbl[])
          }
        }
      }
      frame "Stop" {
      }
    }
    n309 = local read "Quit"() -> (w704:bool)
    n310 = Not(x=w704) -> (.not. x?=w698:bool)
  }
  n311 = while {
    tunnel: w8 -> [_]
    tunnel: [w755] -> w7
    stop <- w755 stop-if-true
    n312 = local read "Load Cell \nReading"() -> (w759:dbl[])
    "Load Cell \nReading  GUI" <- w759
    n313 = local read "LVDT Reading"() -> (w760:dbl[])
    "LVDT Reading  GUI" <- w760
    n314 = local read "Servo Error Reading"() -> (w758:dbl[])
    "Servo Error Reading GUI" <- w758
    n315 = local read "Cal Sensor"() -> (→"Cal Sensor GUI":dbl[])
    n316 = local read "Readings"() -> (w763:T13)
    n317 = case shown="\"LVDT\"" w763 {
      tunnel: w760 -> [w764 _ _]
      tunnel: w759 -> [_ w765 _]
      tunnel: w758 -> [_ _ w766]
      tunnel: [w764 w765 w766] -> w762
      frame "LVDT" {
      }
      frame "Load Cell" {
      }
      frame "Servo Errors" {
      }
    }
    n318 = Array To Cluster(array=w762) -> (cluster=→"Readings":T23)
    n319 = local read "Quit"() -> (w756:bool)
    n320 = Wait Until Next ms Multiple(millisecond multiple=u32 200) -> ()  [unwired: 1 out]
    n321 = Not(x=w756) -> (.not. x?=w755:bool)
  }
  n322 = Compound Arithmetic op=AND(w7, w29, w41, w43, w39, w32, w21, w17, w6) -> (w42:bool)
  n323 = Not(x=w42) -> (.not. x?=w40:bool)
  n324 = flat-sequence {
    tunnel: w40 -> [w768]
    frame #0 {
      n325 = control-ref of="This VI"() -> (w767:refnum<vi>)
      n326 = local write "Quit"(w768) -> ()
      n327 = disable-structure shown="Disabled" {
        disable-tunnel: w767 -> [w769 _]
        frame Disabled {
          n328 = invoke class="VI" method="FP.Close"(reference=w769) -> ()  [unwired: 2 in, 3 out]
        }
        frame Enabled {
        }
      }
    }
  }
  n329 = call "DAQ Finite Read Servo Errors.vi"("error in"=w37, "Action"=DAQ_Read_Actions."Stop") -> ("error out"=→"Write error out":errorcluster)  [unwired: 3 in, 6 out]
